vi "Motor Move.vi"(7 "Output Port (All Ports)":T2=3 items=["Port A"=0, "Port B"=1, "Port C"=2, "Ports A & B"=4, "Ports A & C"=5, "Ports B & C"=6, "All Ports"=3], 8 "Angle of Rotation (360)":i32=360, 9 "Power (75)":i32=75, 11 "NXT/EV3 2":T1) -> (3 "NXT/EV3":T1)   [LabVIEW 2013]
uses:
  <vilib>/NXT/Subs/MotorOutput.ctl
  <vilib>/NXT/Subs/LVHSConnector.ctl
  <vilib>/NXT/LegoClasses/BrickReference/BrickReference.lvclass
  <vilib>/NXT/LegoClasses/MINDSTORMS/MINDSTORMS.lvclass
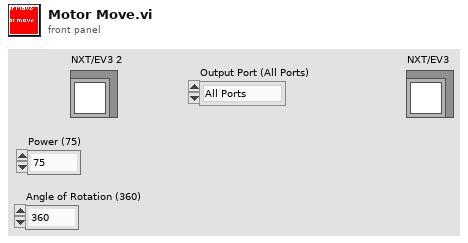
[diagram p1: front panel]
types:
  T1 = typedef "LVHSConnector.ctl" = refnum<class "BrickReference.lvclass">
  T2 = typedef "MotorOutput.ctl" = u8
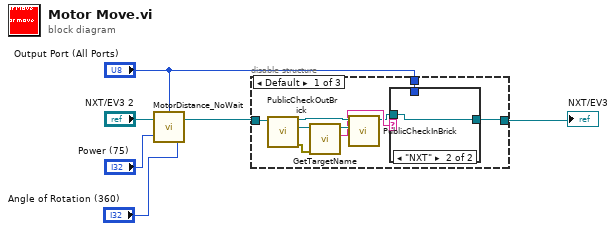
[diagram p0: block diagram]
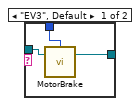
[diagram p2: hidden frame]
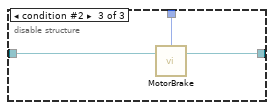
[diagram p4: hidden frame]
diagram:
  n1 = call <vilib>:"MotorDistance_NoWait.vi"("Power (75)"="Power (75)", "Angle of Rotation (360)"="Angle of Rotation (360)", "NXT/EV3"="NXT/EV3 2", "Output Port (All Ports)"="Output Port (All Ports)") -> ("NXT/EV3"=w1:T1)
  n2 = disable-structure shown="Default" {
    disable-tunnel: w1 -> [w15 w20 w21]
    disable-tunnel: "Output Port (All Ports)" -> [w9 _ w23]
    disable-tunnel: [w7 w20 w22] -> w2
    frame condition #0 (active) {
      n3 = call <vilib>:"PublicCheckOutBrick.vi"("BrickReference in"=w15) -> ("error out"=w14:errorcluster, "MINDSTORMS.lvclass"=w13:refnum<class "MINDSTORMS.lvclass">, "BrickReference out"=w12:refnum<class "BrickReference.lvclass">)  [unwired: 8 in]
      n4 = call-dynamic "GetTargetName.vi"("error in (no error)"=w14, "MINDSTORMS in"=w13) -> ("TargetName"=w10:string, "MINDSTORMS out"=w11:refnum<class "MINDSTORMS.lvclass">)  [unwired: 7 in, 1 out]
      n5 = call <vilib>:"PublicCheckInBrick.vi"("MINDSTORMS"=w11, "BrickReference in"=w12) -> ("BrickReference out"=w8:refnum<class "BrickReference.lvclass">)  [unwired: 8 in, 1 out]
      n6 = case shown="\"NXT\"" w10 {
        tunnel: w9 -> [w18 _]
        tunnel: w8 -> [w17 w19]
        tunnel: [w16 w19] -> w7
        frame "EV3", Default {
          n7 = call <vilib>:"MotorBrake.vi"("NXT/EV3"=w17, "Port (All Ports)"=w18) -> ("NXT/EV3"=w16:T1)  [unwired: 2 in]
        }
        frame "NXT" {
        }
      }
    }
    frame condition #1 {
    }
    frame condition #2 {
      n8 = call <vilib>:"MotorBrake.vi"("NXT/EV3"=w21, "Port (All Ports)"=w23) -> ("NXT/EV3"=w22:T1)  [unwired: 2 in]
    }
  }
  "NXT/EV3" <- w2
